vi "Create.vi"(8 "error in (no error)":errorcluster, 11 "U16 array in":u16[](array[numeric])) -> (0 "error out":errorcluster, 3 "Uint16Array out":refnum<class "Uint16Array.lvclass">)   [LabVIEW 2012, in "MDSplus.lvlib" / "Uint16Array.lvclass"]
uses:
  <vilib>/MDSplus/Classes/Data_Class/Array_Class/Uint16Array_Class/Uint16Array.lvclass
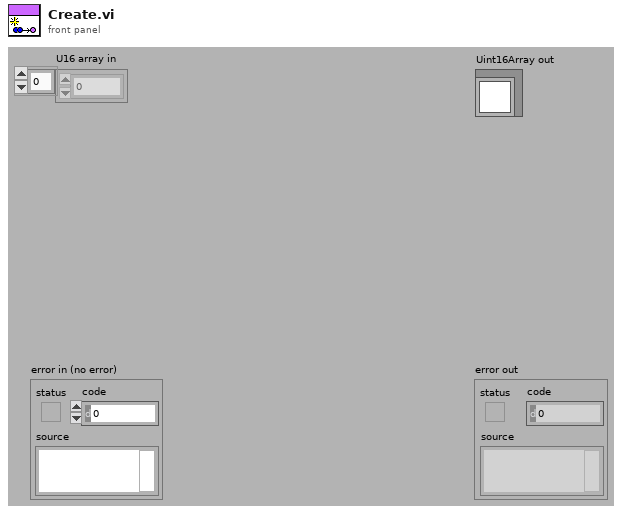
[diagram p1: front panel]
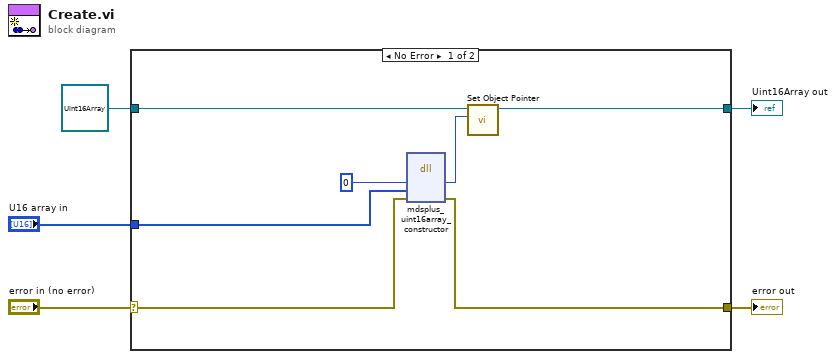
[diagram p0: block diagram]
diagram:
  n1 = case shown="No Error" "error in (no error)" {
    selector: "error in (no error)" -> [w10 w14]
    tunnel: [w6 w14] -> w4
    tunnel: [w8 w13] -> w2
    tunnel: refnum<class "Uint16Array.lvclass"> refnum ("Float32 in") -> [w9 w13]
    tunnel: "U16 array in" -> [w7 _]
    frame No Error {
      n2 = dll-call lib="MDSobjectsLVShr" fn="mdsplus_uint16array_constructor"("lvUint16ArrayPtrOut"=i64 0 ("lvTreePtr"), "lvUShtArrHdlIn"=w7, "error"=w10) -> ("lvUint16ArrayPtrOut"=w11:i64, "error"=w6:errorcluster)  [unwired: 5 in, 2 out]
      n3 = call-dynamic "Set Object Pointer.vi"("Object Pointer"=w11, "Data in"=w9) -> ("Data out"=w8:refnum<class "Uint16Array.lvclass">)  [unwired: 9 in]
    }
    frame Error {
    }
  }
  "error out" <- w4
  "Uint16Array out" <- w2
